vi "Erase Comments.vi"(8 "error in (no error)":errorcluster, 11 "AFM Control":refnum<class "AFM Control.lvclass">) -> (0 "error out":errorcluster, 3 "AFM Control out":refnum<class "AFM Control.lvclass">)   [LabVIEW 2020, in "AFM Control.lvclass"]
uses:
  AFM Control.lvclass
  AFM Control.lvclass/AFM Control.ctl
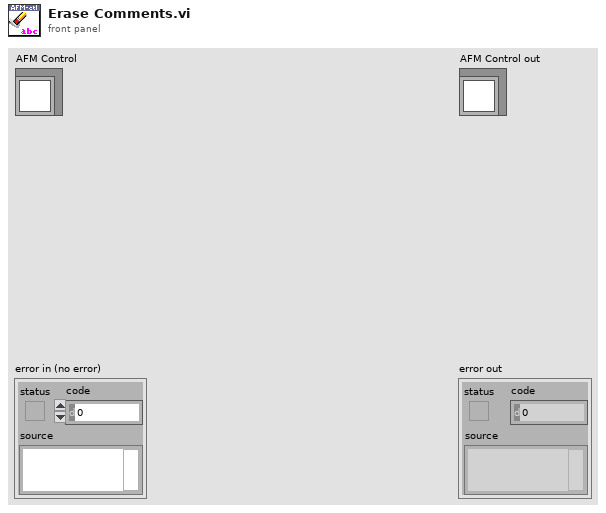
[diagram p1: front panel]
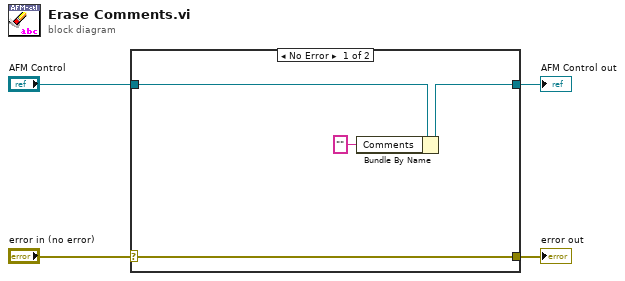
[diagram p0: block diagram]
diagram:
  n1 = case shown="No Error" "error in (no error)" {
    selector: "error in (no error)" -> [w8 w9]
    tunnel: [w8 w9] -> w3
    tunnel: [w6 w10] -> w1
    tunnel: "AFM Control" -> [w7 w10]
    frame No Error {
      n2 = Bundle By Name(cluster=w7, "Comments"="") -> (w6:refnum<class "AFM Control.lvclass">)
    }
    frame Error {
    }
  }
  "error out" <- w3
  "AFM Control out" <- w1
